vi "SwitchBlock Arrays.vi"(8 "error in (no error)":errorcluster, 9 "Number of Rows":i32, 10 "Number of Cards":i32) -> (0 "error out":errorcluster, 1 "Analog Bus Array":string[](array[string]), 2 "Row Array":string[](array[string]))   [LabVIEW 2019]
doc: "I. Description:\n\nThis is a subVI for use with NI Switchblock. This VI takes in the number of cards and rows on your NI SwitchBlock device and outputs two arrays filled with the names of the rows and analog buses on your NI SwitchBlock Device.\n\nII. Instructions for Running:\n\n1. Select the number of cards and rows on your NI SwitchBlock device. \n2. Then hit run, and a list will be generated showing all rows and analog buses available.\n\nRefer to the NI Switches Help for the valid channel names for your switch module.\n\nIII. Block Diagram Steps:\n\n1. This first For Loop iterates through the number of cards on your NI SwitchBlock device, it converts the iteration number and appends this information to begin the creation of the Row Array.\n2. The second For Loop iterates through the number of rows on each card of your NI SwitchBlock device, it converts the iteration number and appends this information to complete the entire string row name.\n3. This builds the Row Array with each row's individual name that has been created in the previous steps.\n4. This For Loop creates the Analog Bus Array based on the number of rows."
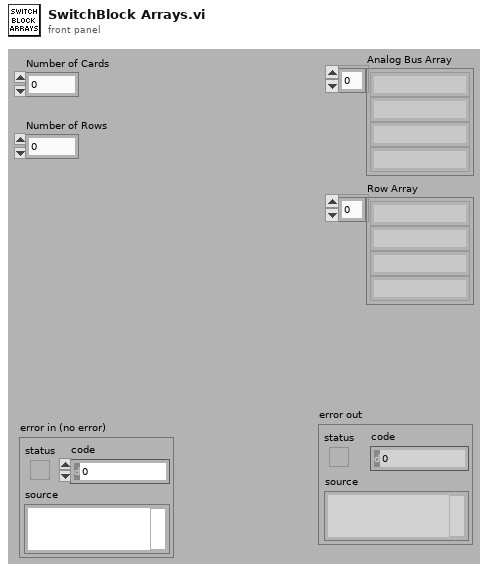
[diagram p1: front panel]
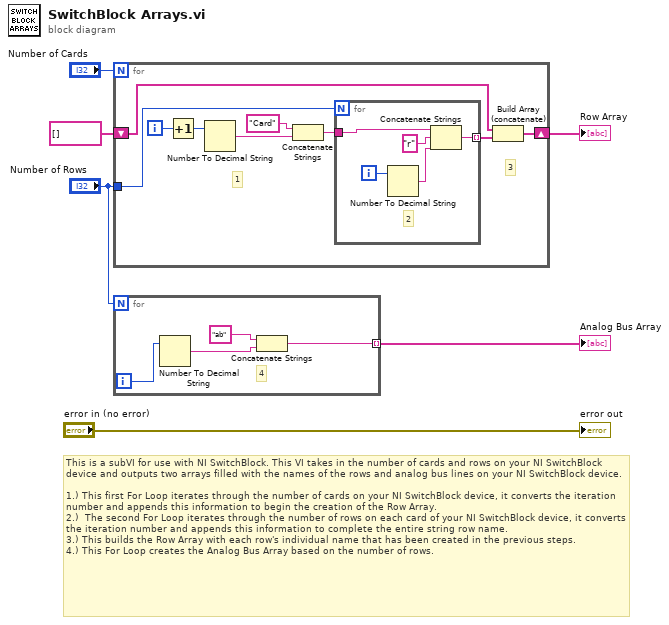
[diagram p0: block diagram]
diagram:
  # "This is a subVI for use with NI SwitchBlock. This VI takes in the number of cards and rows on your NI SwitchBlock device and outputs two arrays filled with the names of the rows and analog bus lines on your NI SwitchBlock device.\n\n1.) This first For Loop iterates through the number of cards on your NI SwitchBlock device, it converts the iteration number and appends this information to begin the creation of the Row Array.\n2.)  The second For Loop iterates through the number of rows on each card of your NI SwitchBlock device, it converts the iteration number and appends this information to complete the entire string row name.\n3.) This builds the Row Array with each row's individual name that has been created in the previous steps.\n4.) This For Loop creates the Analog Bus Array based on the number of rows."
  n1 = for {
    N: "Number of Cards" -> [_]
    tunnel: "Number of Rows" -> [w10]
    shift-right: [w7] -> w6
    shift-left: string[] [] -> [w9]
    i -> [w14]
    # "3"
    # "1"
    n2 = Increment(x=w14) -> (x+1=w13:i32)
    n3 = Number To Decimal String(number=w13) -> (decimal integer string=w12:string)  [unwired: 1 in]
    n4 = Concatenate Strings("Card", w12) -> (w11:string)
    n5 = for {
      N: w10 -> [_]
      tunnel: w11 -> [w19]
      tunnel: [w16] -> w8 mode=indexing
      i -> [w20]
      # "2"
      n6 = Number To Decimal String(number=w20) -> (decimal integer string=w18:string)  [unwired: 1 in]
      n7 = Concatenate Strings(w19, "r" ("string"), w18) -> (w16:string)
    }
    n8 = Build Array (concatenate)(w9, w8) -> (w7:string[])
  }
  "Row Array" <- w6
  n9 = for {
    N: "Number of Rows" -> [_]
    tunnel: [w21] -> w2 mode=indexing
    i -> [w22]
    # "4"
    n10 = Number To Decimal String(number=w22) -> (decimal integer string=w23:string)  [unwired: 1 in]
    n11 = Concatenate Strings("ab", w23) -> (w21:string)
  }
  "Analog Bus Array" <- w2
  "error out" <- "error in (no error)"
